vi "Convert Lat Lon to XY.vi"(11 "Weed Locations (Lat Lon)":T2[](array[typedef]) {"Longitude" format="%#.8g"; "Latitude" format="%#.8g"}) -> (3 "Weed Locations (X & Y)":T1[](array[typedef]) {"Y Coordinate" format="%#_10g"; "X Coordinate" format="%#_10g"})   [LabVIEW 2014]
uses:
  Images/Proccess Images/Contols/Detected Lat Lon.ctl
  Control/SHX Point Data.ctl
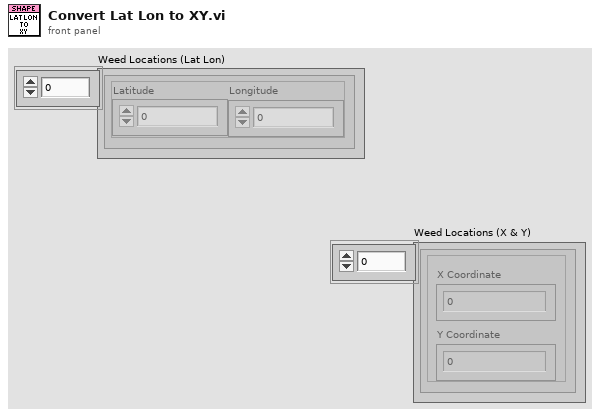
[diagram p1: front panel]
types:
  T1 = typedef "SHX Point Data.ctl" = cluster{"X Coordinate":dbl, "Y Coordinate":dbl}
  T2 = typedef "Detected Lat Lon.ctl" = cluster{"Latitude":dbl, "Longitude\n":dbl}
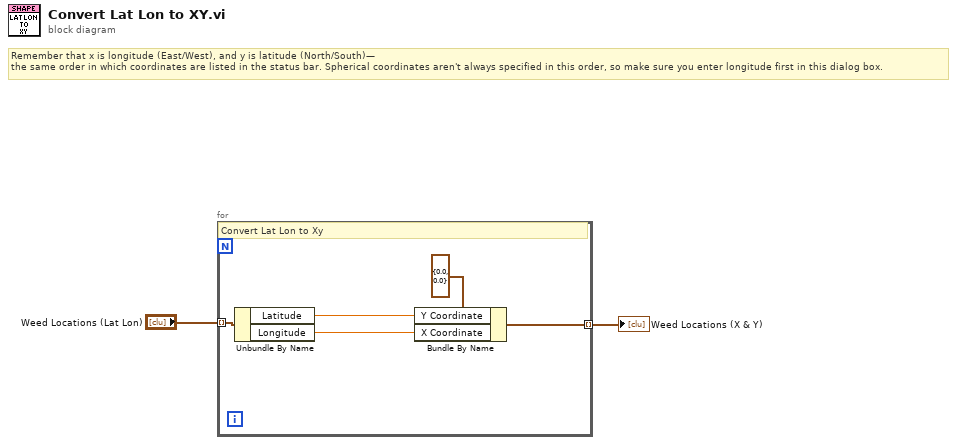
[diagram p0: block diagram]
diagram:
  # "Remember that x is longitude (East/West), and y is latitude (North/South)—\nthe same order in which coordinates are listed in the status bar. Spherical coordinates aren't always specified in this order, so make sure you enter longitude first in this dialog box."
  n1 = for {
    tunnel: "Weed Locations (Lat Lon)" -> [w7] mode=indexing
    tunnel: [w3] -> w1 mode=indexing
    # "Convert Lat Lon to Xy"
    n2 = Unbundle By Name(w7) -> ("Latitude"=w5:dbl, "Longitude"=w4:dbl)
    n3 = Bundle By Name(cluster=T1 {"X Coordinate"=0.0, "Y Coordinate"=0.0} ("SHX Point"), "Y Coordinate"=w5, "X Coordinate"=w4) -> (w3:T1)
  }
  "Weed Locations (X & Y)" <- w1
